vi "LaserParameterSetGetFGV.vi"(8 "error in":errorcluster) -> (0 "error out":errorcluster)   [LabVIEW 2010]
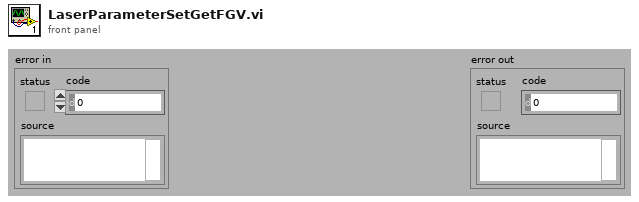
[diagram p1: front panel]
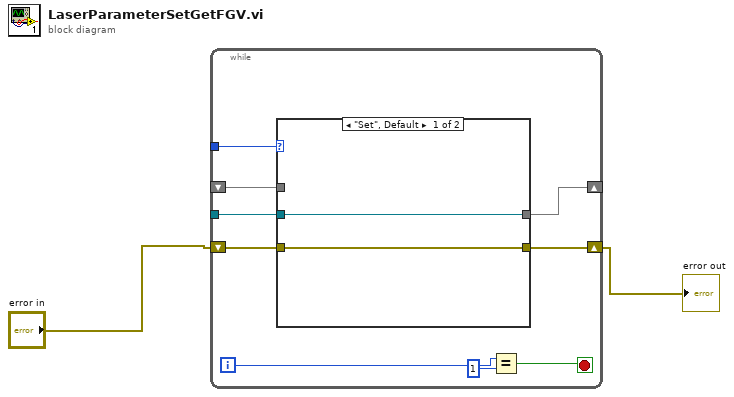
[diagram p0: block diagram]
diagram:
  n1 = while {
    tunnel: [w14] -> w5
    tunnel: [w13] -> w4
    shift-right: [w12] -> w3
    shift-left: _ -> [w11]
    shift-right: [w6] -> w1
    shift-left: "error in" -> [w7]
    i -> [w9]
    stop <- w10 stop-if-true
    n2 = case shown="\"Set\", Default" w14 {
      tunnel: w13 -> [w16 _]
      tunnel: [w16 w18] -> w12
      tunnel: w11 -> [_ w18]
      tunnel: w7 -> [w15 w17]
      tunnel: [w15 w17] -> w6
      frame "Set", Default {
      }
      frame "Get" {
      }
    }
    n3 = Equal?(x=w9, y=1) -> (x = y?=w10:bool)
  }
  "error out" <- w1
